vi "Set State_Measure iVIO only.vi"(0 "Semiconductor Module Context":T1, 1 "script name":string, 2 "Delay Time (s)":dbl=0.001 format="%#_13p", 7 "Power_Pins":string[](array[string]), 9 "Published Data Ids":string[](array[string]), 11 "error in (no error)":errorcluster) -> (15 "error out":errorcluster)   [LabVIEW 2013]
uses:
  <vilib>/NI_TestStand_SemiconductorModule/NI_TestStand_Semiconductor_Module.lvlibp/PinMap/General/SemiconductorModuleContext.ctl
  <instrlib>/niHSDIO/niHSDIO.llb/niHSDIO_ctl Trigger Script - trigID Values (Ring).ctl
  <vilib>/NI_TestStand_SemiconductorModule/NI_TestStand_Semiconductor_Module.lvlibp/PinMap/DC Power/PinsToNIDCPowerSessions.vi
  <vilib>/NI_TestStand_SemiconductorModule/NI_TestStand_Semiconductor_Module.lvlibp/PinMap/General/Publish/PublishDataDouble2D.vi
  <vilib>/NI_TestStand_SemiconductorModule/NI_TestStand_Semiconductor_Module.lvlibp
panel:
  out "current measurements":dbl[][](array[numeric])
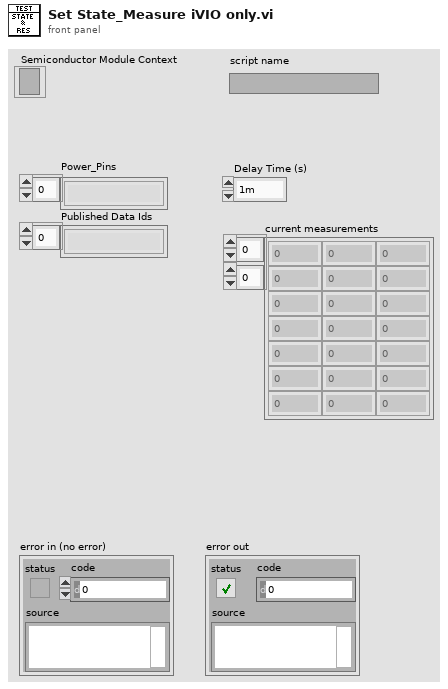
[diagram p1: front panel]
types:
  T1 = typedef "NI_TestStand_Semiconductor_Module.lvlibp/SemiconductorModuleContext.ctl" = refnum<k7>
  T2 = typedef "niHSDIO_ctl Trigger Script - trigID Values (Ring).ctl" = string
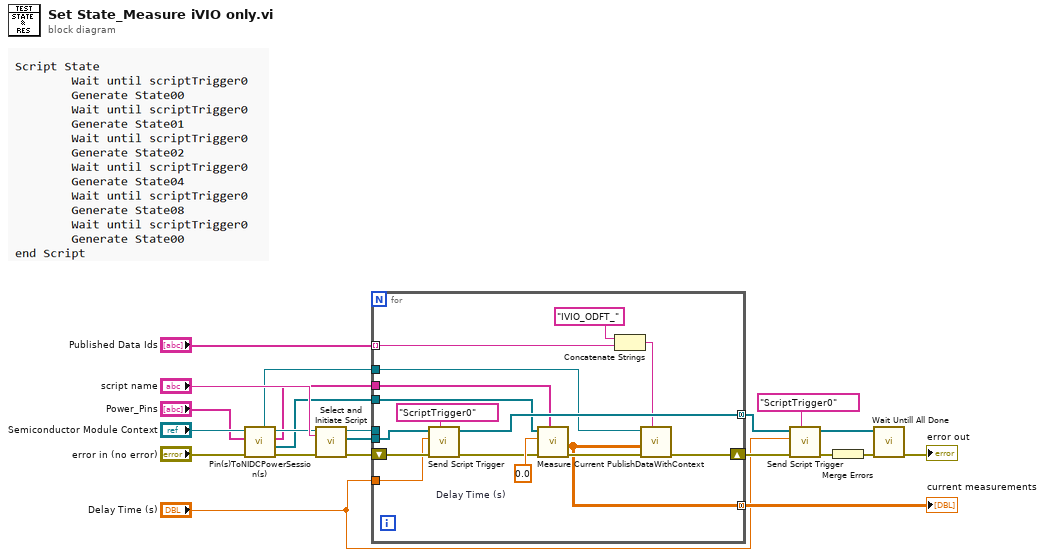
[diagram p0: block diagram]
diagram:
  n1 = call-poly <vilib>:"Pin(s)ToNIDCPowerSession(s).vi"("error in (no error)"="error in (no error)", "Pins"="Power_Pins", "Semiconductor Module Context"="Semiconductor Module Context") -> ("error out"=w11:errorcluster, "Instrument Sessions"=w6:refnum<k15>[], "Channel Lists"=w5:string[], "Semiconductor Module Context Out"=w8:T1, "Pin Query Context"=w3:refnum<class "MultiplePinMultipleSessionQueryContext.lvclass">)  [unwired: 4 in]
  n2 = call "Select and Initiate Script.vi"("error in (no error)"=w11, "script name"="script name", "Semiconductor Module Context"=w8) -> ("error out"=w22:errorcluster, "HSDIO GEN Sessions Out"=w21:refnum<k15>[], "Semiconductor Module Context Out"=w19:T1)  [unwired: 6 in]
  n3 = for {
    tunnel: w21 -> [w37]
    tunnel: w19 -> [_]
    tunnel: "Published Data Ids" -> [w27] mode=indexing
    tunnel: [w35] -> w13 mode=concatenating
    shift-right: [w30] -> w4
    shift-left: w22 -> [w38]
    tunnel: w6 -> [w32]
    tunnel: w5 -> [w33]
    tunnel: w3 -> [w29]
    tunnel: [w28] -> w2 mode=concatenating
    tunnel: "Delay Time (s)" -> [w23]
    w34 = 0.0  # Delay Time (s)
    n4 = call "Send Script Trigger.vi"("trigger id (script trigger 0)"=T2 "ScriptTrigger0", "error in (no error)"=w38, "Delay Time (s)"=w23, "HSDIO Sessions In"=w37) -> ("error out"=w24:errorcluster, "HSDIO Sessions Out"=w35:refnum<k15>[])  [unwired: 6 in]
    n5 = call "Measure Current.vi"("Channel Lists"=w33, "error in (no error)"=w24, "Delay Time (s)"=w34, "DCPower Sessions In"=w32) -> ("error out"=w31:errorcluster, "current measurements"=w28:dbl[][])  [unwired: 5 in, 1 out]
    n6 = Concatenate Strings("IVIO_ODFT_" ("Published Data Id"), w27) -> (w26:string)
    n7 = call-poly <vilib>:"PublishDataWithContext.vi"("Published Data Id"=w26, "error in (no error)"=w31, "Data In"=w28, "Pin Query Context"=w29) -> ("error out"=w30:errorcluster)  [unwired: 6 in, 1 out]
  }
  "current measurements" <- w2
  n8 = call "Send Script Trigger.vi"("trigger id (script trigger 0)"=T2 "ScriptTrigger0", "error in (no error)"=w4, "Delay Time (s)"="Delay Time (s)", "HSDIO Sessions In"=w13) -> ("error out"=w14:errorcluster, "HSDIO Sessions Out"=w12:refnum<k15>[])  [unwired: 6 in]
  n9 = Merge Errors(w14) -> (w17:errorcluster)
  n10 = call "Wait Untill All Done.vi"("error in (no error)"=w17, "HSDIO Sessions In"=w12) -> ("error out"=→"error out":errorcluster)  [unwired: 8 in, 1 out]
